vi "Ejercicio_2_4.vi"() -> ()   [LabVIEW 2020]
panel:
  out "Resultado":string
  out "?":string
  out "?":string
  out "?":string
  out "?":string
  in  "Operaciones":i32(slide) scale=0.0..3.0
  in  "Numero 2":dbl
  in  "Numero 1":dbl
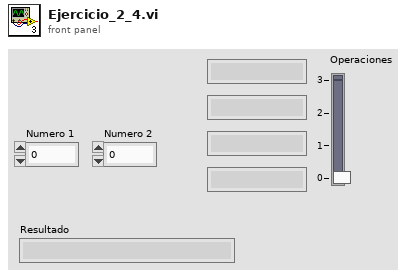
[diagram p1: front panel]
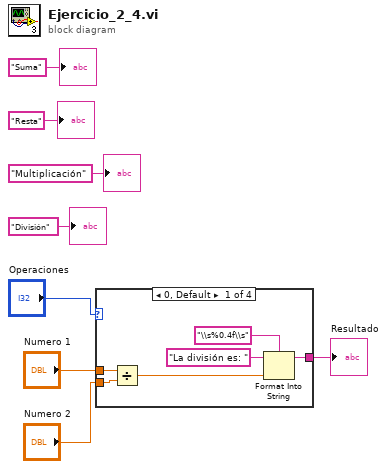
[diagram p0: block diagram]
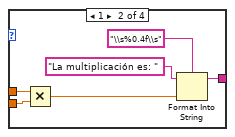
[diagram p2: hidden frame]
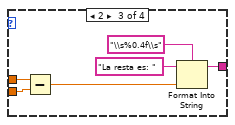
[diagram p3: hidden frame]
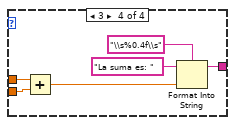
[diagram p4: hidden frame]
diagram:
  n1 = case shown="0, Default" "Operaciones" {
    tunnel: "Numero 1" -> [w14 w20 w26 w32]
    tunnel: "Numero 2" -> [w13 w19 w25 w31]
    tunnel: [w9 w15 w21 w27] -> w1
    frame 0, Default {
      n2 = Divide(x=w14, y=w13) -> (x/y=w10:dbl)
      n3 = Format Into String(format string="\\s%0.4f\\s", initial string="La división es: ", w10) -> (resulting string=w9:string)  [unwired: 1 in, 1 out]
    }
    frame 1 {
      n4 = Multiply(x=w20, y=w19) -> (x*y=w16:dbl)
      n5 = Format Into String(format string="\\s%0.4f\\s", initial string="La multiplicación es: ", w16) -> (resulting string=w15:string)  [unwired: 1 in, 1 out]
    }
    frame 2 {
      n6 = Subtract(x=w26, y=w25) -> (x-y=w22:dbl)
      n7 = Format Into String(format string="\\s%0.4f\\s", initial string="La resta es: ", w22) -> (resulting string=w21:string)  [unwired: 1 in, 1 out]
    }
    frame 3 {
      n8 = Add(x=w32, y=w31) -> (x+y=w30:dbl)
      n9 = Format Into String(format string="\\s%0.4f\\s", initial string="La suma es: ", w30) -> (resulting string=w27:string)  [unwired: 1 in, 1 out]
    }
  }
  "Resultado" <- w1
  "?" <- "Suma"
  "?" <- "Resta"
  "?" <- "Multiplicación"
  "?" <- "División"
